vi "AO Control.vi"(4 "pause/resume channel list (empty)":string[](array[string])=[""], 6 "iterations (0: infinite)":i32, 8 "error in (no error)":errorcluster, 9 "staging list (empty)":T1(array[cluster]) {"ARB mode:  marker offset\nDDS mode:  output freq. (Hz)" format="%0.2f"}, 10 "control code (0: start)":u16(ring) items=["start", "pause", "pause at EOC", "resume", "clear", "switch to next buffer", "switch to next buffer at EOC", "new staging list"], 11 "task ID":u32 format="%x") -> (0 "error out":errorcluster, 3 "task ID out":u32 format="%x")   [LabVIEW 2009]
doc: "Starts, pauses, resumes, and clears analog output tasks."
uses:
  <vilib>/Daq/lvdaq.dll
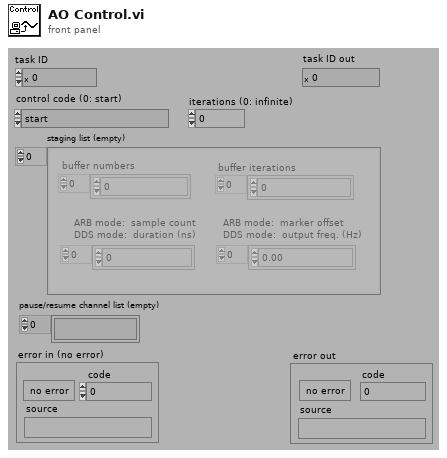
[diagram p1: front panel]
types:
  T1 = cluster{"buffer numbers":i32[], "buffer iterations":i32[], "ARB mode:  sample count\nDDS mode:  duration (ns)":i32[], "ARB mode:  marker offset\nDDS mode:  output freq. (Hz)":dbl[]}[]
  T2 = enum16{"start", "pause", "pause at EOC", "resume", "clear", "switch to next buffer", "switch to next buffer at EOC"}
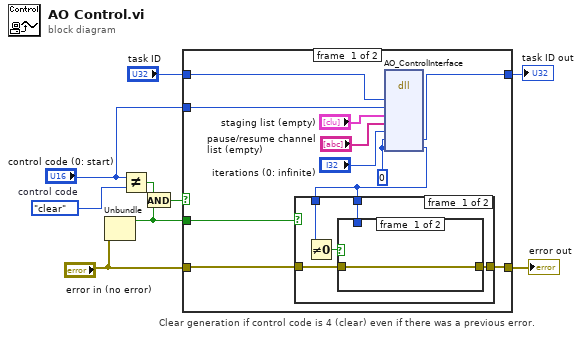
[diagram p0: block diagram]
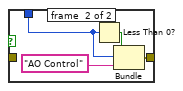
[diagram p2: hidden frame]
diagram:
  w1 = T2."clear"  # control code
  # "Clear generation if control code is 4 (clear) even if there was a previous error."
  n1 = Unbundle("error in (no error)") -> ("status"=w2:bool)  [unwired: 2 out]
  n2 = Not Equal?(x="control code (0: start)", y=w1) -> (x != y?=w4:bool)
  n3 = And(x=w4, y=w2) -> (x .and. y?=w3:bool)
  n4 = case shown="False" w3 {
    tunnel: [w12 w32] -> w7
    tunnel: "task ID" -> [w17 w33]
    tunnel: [w16 w33] -> w8
    tunnel: "error in (no error)" -> [w11 w32]
    tunnel: "control code (0: start)" -> [w15 _]
    tunnel: w2 -> [w14 _]
    frame #0 {
      w18 = 0
      n5 = dll-call lib="C:/Program Files/National Instruments/LabVIEW 2009/vi.lib/Daq/lvdaq.*" fn="AO_ControlInterface"(w17, w15, "staging list (empty)", "pause/resume channel list (empty)", "iterations (0: infinite)", w18, w18) -> (w16:i32, w13:i32)  [unwired: 9 in, 2 out]
      n6 = case shown="False" w14 {
        tunnel: w13 -> [w25 _]
        tunnel: w13 -> [w23 _]
        tunnel: [w22 w31] -> w12
        tunnel: w11 -> [w21 w31]
        frame #0 {
          n7 = Not Equal To 0?(x=w25) -> (x != 0?=w24:bool)
          n8 = case shown="True" w24 {
            tunnel: w23 -> [_ w29]
            tunnel: [w26 w27] -> w22
            tunnel: w21 -> [w26 _]
            frame #0 {
            }
            frame #1 {
              n9 = Less Than 0?(x=w29) -> (x < 0?=w30:bool)
              n10 = Bundle(w30, w29, "AO Control") -> (w27:errorcluster)  [unwired: 1 in]
            }
          }
        }
        frame #1 {
        }
      }
    }
    frame #1 {
    }
  }
  "task ID out" <- w8
  "error out" <- w7
